vi "Ball Index (SubVI).vi"(9 "Ball index":i32, 10 "reference in":refnum<vi>, 11 "Digital in":refnum<vi>) -> ()   [LabVIEW 2017]
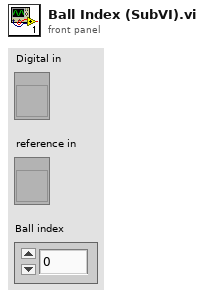
[diagram p1: front panel]
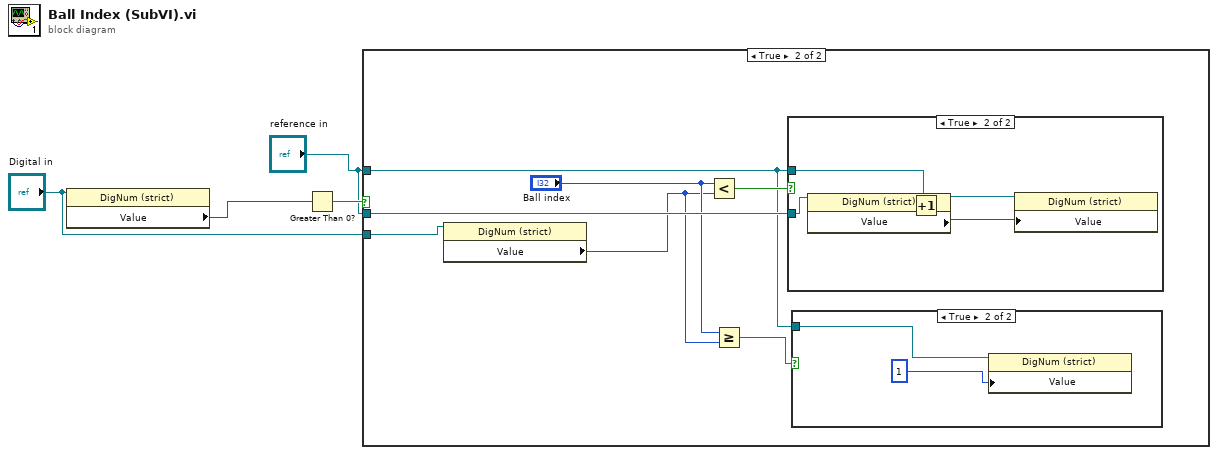
[diagram p0: block diagram]
diagram:
  n1 = property class="DigNum (strict)"(reference="Digital in") -> ("Value"=w3:i32)  [unwired: 1 in, 2 out]
  n2 = Greater Than 0?(x=w3) -> (x > 0?=w4:bool)
  n3 = case shown="True" w4 {
    tunnel: "reference in" -> [_ w5]
    tunnel: "reference in" -> [_ w10]
    tunnel: "Digital in" -> [_ w9]
    frame False {
    }
    frame True {
      n4 = property class="DigNum (strict)"(reference=w9) -> ("Value"=w7:i32)  [unwired: 1 in, 2 out]
      n5 = Less?(x="Ball index", y=w7) -> (x < y?=w11:bool)
      n6 = Greater Or Equal?(x="Ball index", y=w7) -> (x >= y?=w6:bool)
      n7 = case shown="True" w11 {
        tunnel: w5 -> [_ w15]
        tunnel: w10 -> [_ w14]
        frame False {
        }
        frame True {
          n8 = property class="DigNum (strict)"(reference=w14) -> ("Value"=w17:i32)  [unwired: 1 in, 2 out]
          n9 = Increment(x=w17) -> (x+1=w16:i32)
          n10 = property class="DigNum (strict)"(reference=w15, "Value"=w16) -> ()  [unwired: 1 in, 2 out]
        }
      }
      n11 = case shown="True" w6 {
        tunnel: w5 -> [_ w13]
        frame False {
        }
        frame True {
          n12 = property class="DigNum (strict)"(reference=w13, "Value"=1 ("Ball index")) -> ()  [unwired: 1 in, 2 out]
        }
      }
    }
  }
